vi "Configure LIST BAND.vi"(5 "High Limit Value (0)":dbl, 6 "Low Limit Value (0)":dbl, 7 "User Parameter (0:OFF)":i32(ring) items=["OFF", "A", "B"], 8 "error in (no error)":errorcluster, 9 "Sweep Point Value (0)":dbl, 10 "List Sweep Point (1)":i32=1 min=1 max=10 step=1, 11 "VISA resource name":refnum<visa-resource-name>) -> (0 "error out":errorcluster, 3 "VISA resource name out":refnum<visa-resource-name>)   [LabVIEW 2014, in "LCR Meter.lvlib"]
doc: "Sets the List Sweep point value, limit mode and low/high limit values."
uses:
  <instrlib>/LCR Meter/Examples/LCR Meter Acquire Single_1 Folder/LCR Meter.lvlib
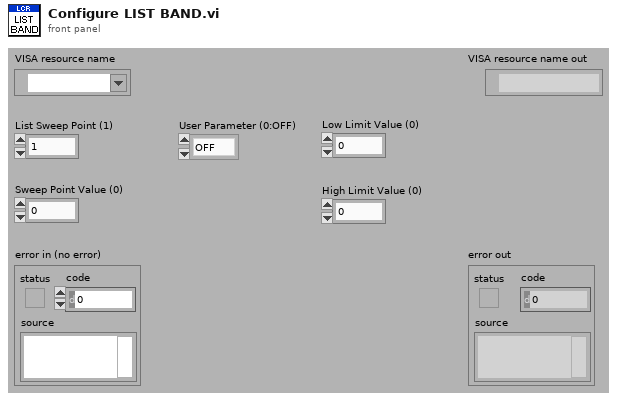
[diagram p1: front panel]
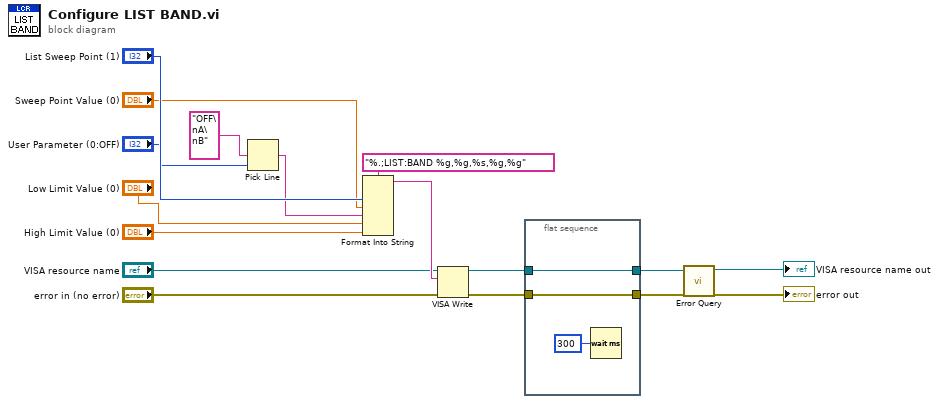
[diagram p0: block diagram]
diagram:
  n1 = Pick Line(multi-line string="OFF\nA\nB", line index="User Parameter (0:OFF)") -> (output string=w5:string)  [unwired: 1 in]
  n2 = Format Into String(format string="%.;LIST:BAND %g,%g,%s,%g,%g", "List Sweep Point (1)", "Sweep Point Value (0)", w5, "Low Limit Value (0)", "High Limit Value (0)") -> (resulting string=w12:string)  [unwired: 2 in, 1 out]
  n3 = VISA Write(VISA resource name="VISA resource name", write buffer=w12, error in (no error)="error in (no error)") -> (VISA resource name out=w4:refnum<visa-resource-name>, error out=w2:errorcluster)  [unwired: 1 out]
  n4 = flat-sequence {
    tunnel: w4 -> [w20]
    tunnel: [w20] -> w3
    tunnel: w2 -> [w19]
    tunnel: [w19] -> w1
    frame #0 {
      n5 = Wait (ms)(milliseconds to wait=u32 300) -> ()  [unwired: 1 out]
    }
  }
  n6 = call <instrlib>:"Error Query.vi"("error in (no error)"=w1, "VISA resource name"=w3) -> ("error out"=→"error out":errorcluster, "VISA resource name out"=→"VISA resource name out":refnum<visa-resource-name>)  [unwired: 6 in, 2 out]
